vi "Arduino Continuous Sampling V2.vi"() -> ()   [LabVIEW 2013, in "LabVIEW Interface for Arduino.lvlib"]
doc: "This VI shows an example of using the continuous aquisition mode on the Arduino to aquire analog input data from a single input pin. The user can set the sample rate for the aquisition when the VI is first run. The maximum aquisition speed of the Arduino is 5KHZ. While this mode is turned on executing other LIFA commands will corrupt analog data. To use other LIFA commands turn continuous mode off first."
uses:
  <vilib>/LabVIEW Interface for Arduino/LabVIEW Interface for Arduino.lvlib
panel:
  out "output array":dbl[](array[numeric])
  in  "Array":dbl[](array[numeric])
  out "Waveform Chart":dbl[](graph)
  in  "Stop":bool
  in  "Sample Rate (HZ)":u16
  in  "Analog Input Pin":u8
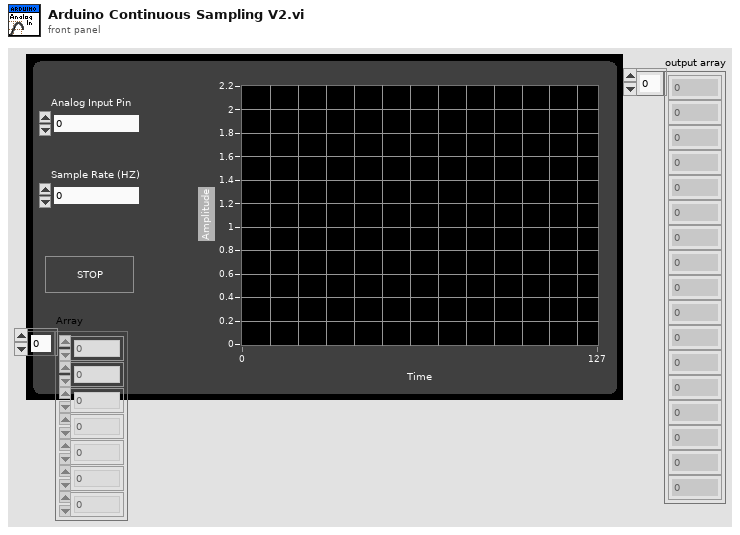
[diagram p1: front panel]
types:
  T1 = typedef "LabVIEW Interface for Arduino.lvlib/Arduino Resource.ctl" = cluster{"VISA resource":refnum<visa-resource-name>, "Board Type":T2, "Connection Type":enum8{"USB / Serial"}, "Bytes Per Packet (15)":u8}
  T2 = typedef "LabVIEW Interface for Arduino.lvlib/Board Type.ctl" = enum16{"Uno", "Dimuelanove w/Atmega 328", "Mega 2560"}
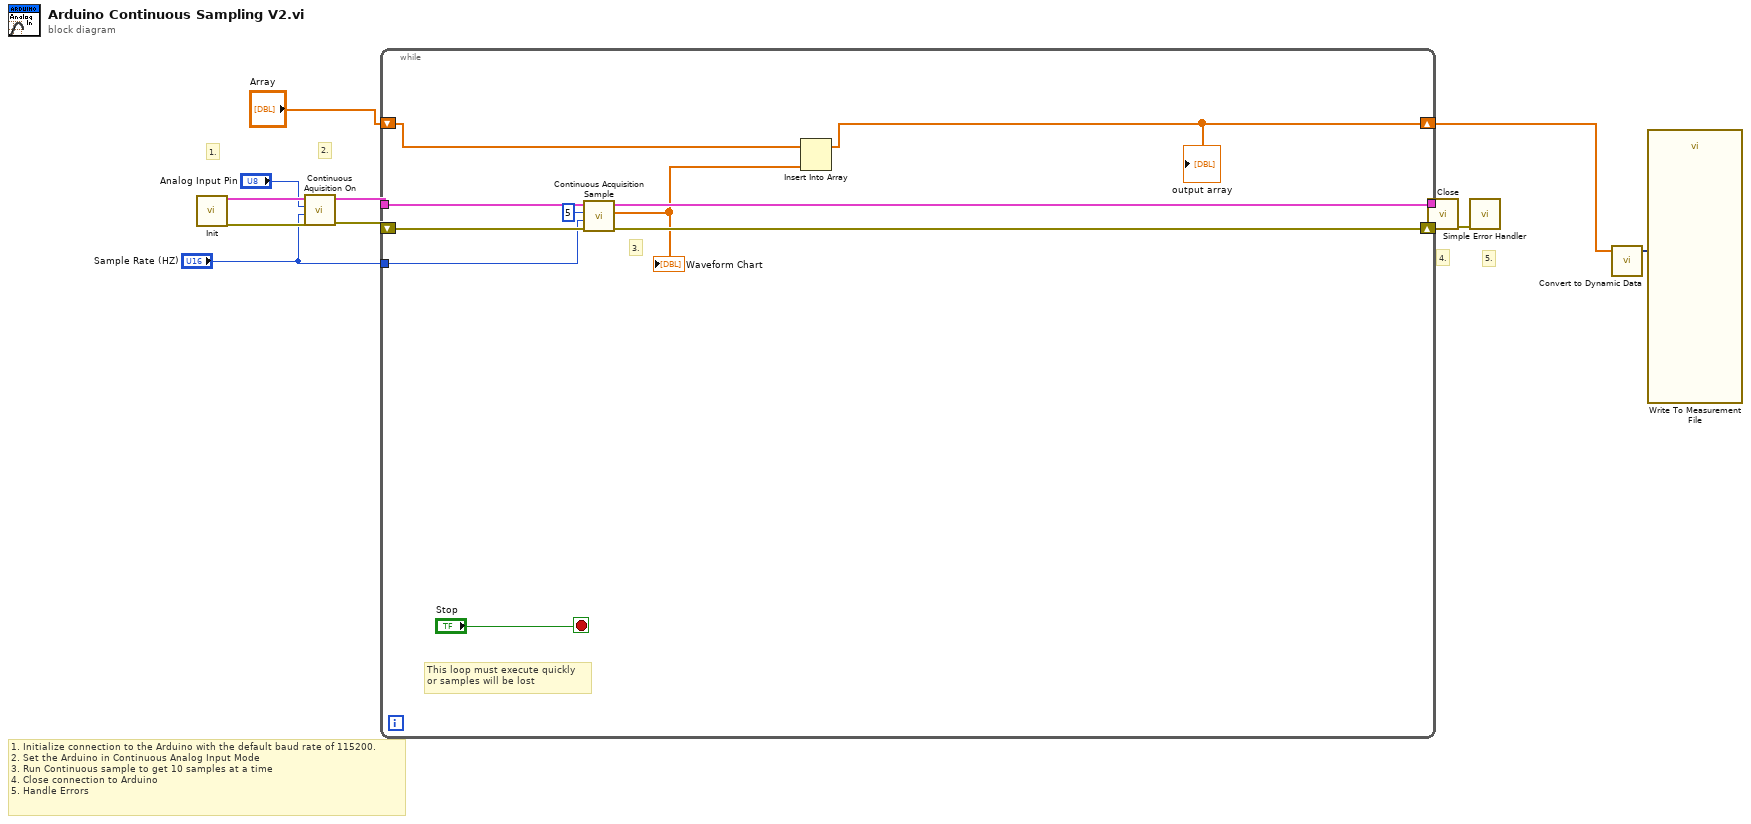
[diagram p0: block diagram]
diagram:
  # "5."
  # "4."
  # "2."
  # "1."
  # "1. Initialize connection to the Arduino with the default baud rate of 115200.\n2. Set the Arduino in Continuous Analog Input Mode\n3. Run Continuous sample to get 10 samples at a time\n4. Close connection to Arduino\n5. Handle Errors"
  n1 = call <vilib>:"Init.vi"() -> ("Arduino Resource"=w12:T1, "error out"=w5:errorcluster)  [unwired: 18 in]
  n2 = call <vilib>:"Continuous Aquisition On.vi"("error in"=w5, "Acquition Speed"="Sample Rate (HZ)", "Analog Input Pin"="Analog Input Pin", "Arduino Resource"=w12) -> ("error out"=w10:errorcluster, "Arduino Resource"=w11:T1)  [unwired: 6 in]
  n3 = while {
    tunnel: w11 -> [w21]
    tunnel: [w20] -> w9
    shift-right: [w19] -> w6
    shift-left: w10 -> [w18]
    tunnel: "Sample Rate (HZ)" -> [w16]
    shift-right: [w13] -> w2
    shift-left: "Array" -> [w15]
    stop <- "Stop" stop-if-true
    # "This loop must execute quickly\nor samples will be lost"
    # "3."
    n4 = call <vilib>:"Continuous Acquisition Sample.vi"("Arduino Resource"=w21, "Samples to Read"=u16 5, "Sample Rate (HZ)"=w16, "error in (no error)"=w18) -> ("Arduino Resource"=w20:T1, "Data"=w14:dbl[], "error out"=w19:errorcluster)  [unwired: 4 in]
    "Waveform Chart" <- w14
    n5 = Insert Into Array(array=w15, new element=w14) -> (w13:dbl[])  [unwired: 1 in]
    "output array" <- w13
  }
  n6 = call <vilib>:"Close.vi"("Arduino Resource"=w9, "error in"=w6) -> ("error out"=w8:errorcluster)  [unwired: 13 in]
  n7 = call <vilib>:"Simple Error Handler.vi"("error in (no error)"=w8) -> ()  [unwired: 4 in, 5 out]
  n8 = call "Convert to Dynamic Data"("Array"=w2) -> ("Dynamic Data Type"=w1:dynamicdata)  [unwired: 3 in]
  n9 = call "Write To Measurement File"("Signals"=w1) -> ()  [unwired: 16 in, 3 out]
